vi "Add Response (Method Not Found).vi"(5 "id value":string, 7 "jsonrpc":string="2.0", 8 "error in (no error)":errorcluster, 10 "data":variant, 11 "Server in":refnum<class "JSONRPC Server.lvclass">) -> (0 "error out":errorcluster, 1 "response string":string, 3 "Server out":refnum<class "JSONRPC Server.lvclass">)   [LabVIEW 2020, in "JSON-RPC Lib.lvlib" / "JSONRPC Server.lvclass"]
uses:
  JSONRPC Server.lvclass
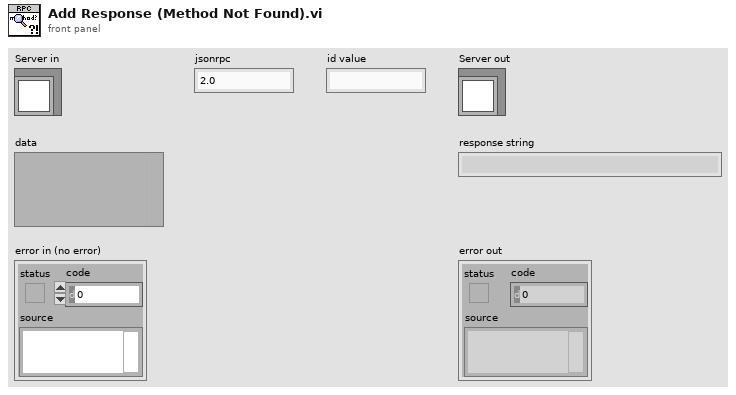
[diagram p1: front panel]
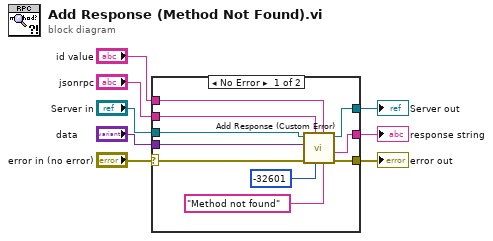
[diagram p0: block diagram]
diagram:
  n1 = case shown="No Error" "error in (no error)" {
    selector: "error in (no error)" -> [w10 w20]
    tunnel: [w11 w20] -> w7
    tunnel: [w17 w19] -> w5
    tunnel: "Server in" -> [w18 w19]
    tunnel: "data" -> [w14 _]
    tunnel: "jsonrpc" -> [w13 _]
    tunnel: "id value" -> [w12 _]
    tunnel: [w9 _] -> w1
    frame No Error {
      n2 = call "Add Response (Custom Error).vi"("message"="Method not found", "id value"=w12, "code"=-32601, "jsonrpc"=w13, "error in (no error)"=w10, "data"=w14, "Server in"=w18) -> ("error out"=w11:errorcluster, "response string"=w9:string, "Server out"=w17:refnum<class "JSONRPC Server.lvclass">)  [unwired: 2 in]
    }
    frame Error {
    }
  }
  "error out" <- w7
  "Server out" <- w5
  "response string" <- w1
